vi "Timer.vi"(7 "Command in":T1, 8 "error in (no error)":errorcluster, 10 "Timer Running?":bool, 11 "Time Limit":i64) -> (0 "error out":errorcluster, 2 "Done?":bool, 3 "Command out":T1)   [LabVIEW 2026]
uses:
  Controls/Timer_Enum.ctl
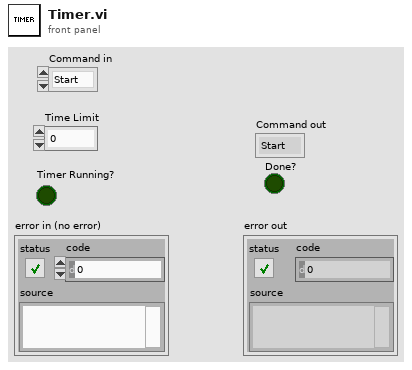
[diagram p1: front panel]
types:
  T1 = typedef "Timer_Enum.ctl" = enum16{"Start", "Read", "Pause", "Stop"}
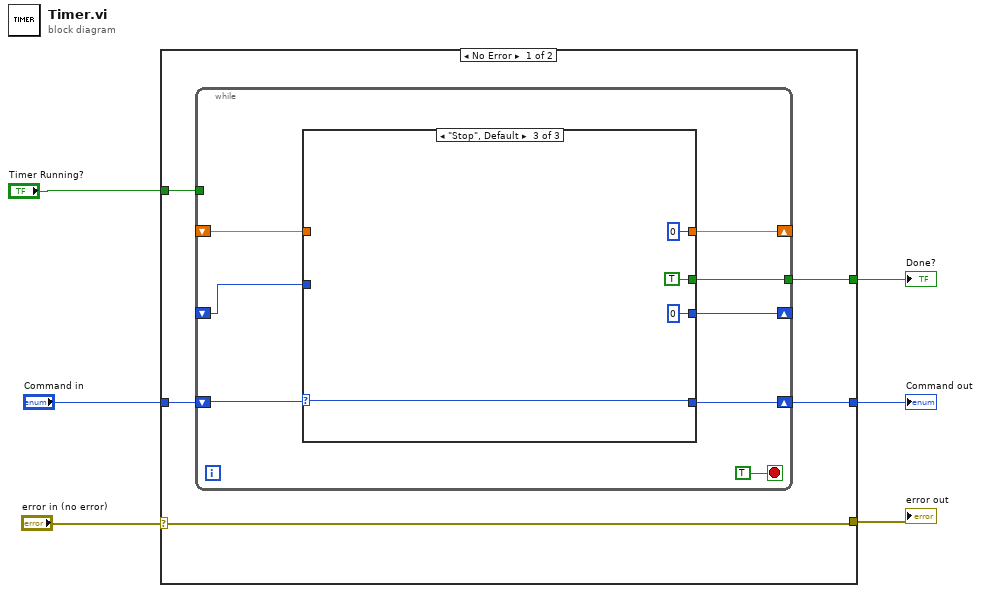
[diagram p0: block diagram]
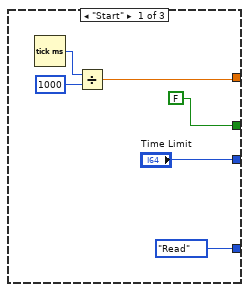
[diagram p2: hidden frame]
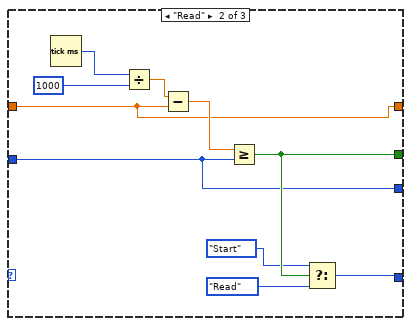
[diagram p3: hidden frame]
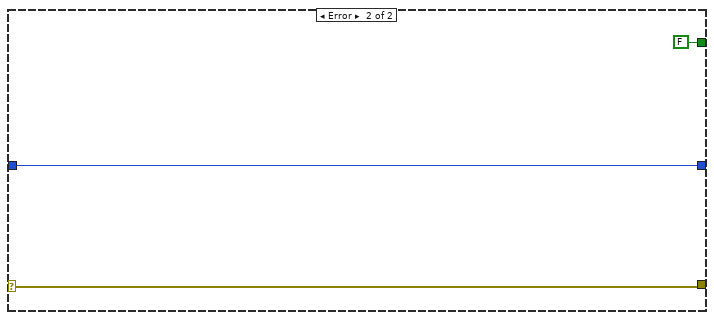
[diagram p4: hidden frame]
diagram:
  n1 = case shown="No Error" "error in (no error)" {
    selector: "error in (no error)" -> [w7 w41]
    tunnel: [w11 w42] -> w6
    tunnel: [w10 FALSE] -> w5
    tunnel: "Timer Running?" -> [w9 _]
    tunnel: "Command in" -> [w8 w42]
    tunnel: [w7 w41] -> w1
    frame No Error {
      n2 = while {
        shift-right: [w17] -> _
        shift-left: _ -> [w15]
        shift-right: [w16] -> w11
        shift-left: w8 -> [w18]
        tunnel: [w14] -> w10
        tunnel: w9 -> [_]
        shift-right: [w13] -> _
        shift-left: _ -> [w12]
        stop <- TRUE stop-if-true
        n3 = case shown="\"Stop\", Default" w18 {
          selector: w18 -> [_ _ w39]
          tunnel: [w21 w27 u32 0 ("millisecond timer value")] -> w17
          tunnel: [Timer_Enum."Read" ("Command in 2") w32 w39] -> w16
          tunnel: w15 -> [_ w27 _]
          tunnel: [FALSE w34 TRUE] -> w14
          tunnel: ["Time Limit" w26 i64 0 ("Time Limit")] -> w13
          tunnel: w12 -> [_ w26 _]
          frame "Start" {
            n4 = Tick Count (ms)() -> (millisecond timer value=w25:u32)
            n5 = Divide(x=w25, y=1000) -> (x/y=w21:dbl)
          }
          frame "Read" {
            n6 = Tick Count (ms)() -> (millisecond timer value=w30:u32)
            n7 = Divide(x=w30, y=u32 1000) -> (x/y=w28:dbl)
            n8 = Subtract(x=w28, y=w27) -> (x-y=w35:dbl)
            n9 = Greater Or Equal?(x=w35, y=w26) -> (x >= y?=w34:bool)
            n10 = Select(t=Timer_Enum."Start" ("Command in 2"), s=w34, f=Timer_Enum."Read" ("Command in 2")) -> (s? t:f=w32:T1)
          }
          frame "Stop", Default {
          }
        }
      }
    }
    frame Error {
    }
  }
  "Command out" <- w6
  "Done?" <- w5
  "error out" <- w1
